vi "cm2nm_add_point_to_list.vi"(0 "SampleDataPoint":T1, 1 "SessionIndex":i32, 3 "Sample locations of Interest":refnum<vi>) -> (2 "sampleOf_interest_duplicate":refnum<vi>)   [LabVIEW 2011]
doc: "add_point_to_list \nadds a sample point to the table whose rows are the unique sample location and the collumns are the sessions. An X in the the row/col combination indicates the sample has been acquired in a particular session. A more complicated variation may be devised later.\n\nif the string associated with the location ID is unique then a new row for this sample will be added to the table and the row labels modified to include this. At this time no sorting will supported but could be added in future revisions.\n\nInputs\nReference to sample locations of Interest Table: reference to the table object on the top level front panel. Passed as a reference so the Row label array can be altered as well as the value of the table locations\n\nSampleDataPoint is the information about the current sample being added to the table. The necessary information is the Location Name/ID. That will be compared to the Row label strings to determine if it existed in prior sessions so it can be assigned to the same row or have a new row created for it.\n\nSessionIndex: number related the session of this data point to the collumn. It is the same index as that stored in the sample data base session lilst.\n\nSampleIndex: number of named samples in the table."
uses:
  cm2nm_coordinate_information_v2.ctl
panel:
  out "size(s)":i32[](array[numeric])
  out "Value":string[][](table)
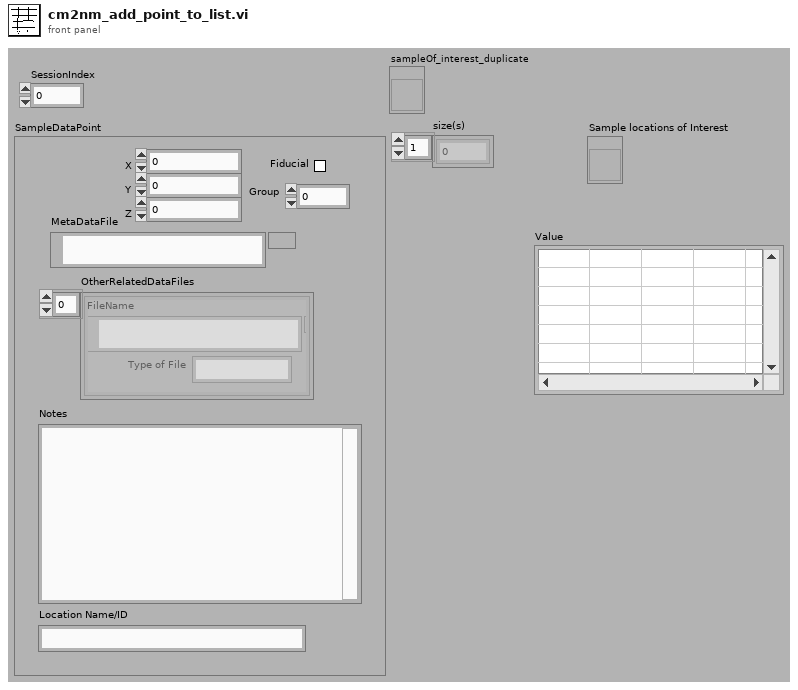
[diagram p1: front panel]
types:
  T1 = typedef "cm2nm_coordinate_information_v2.ctl" = cluster{"MetaDataFile":path, "X":dbl, "Y":dbl, "Z":dbl, "Group":i32, "Rotation":dbl[unit], "Fiducial":bool, "Magnification":dbl, "Working_Distance":dbl, "Notes":string, "Location Name/ID":string, "OtherRelatedDataFiles":cluster{"Type of File":string, "FileName":path}[], "Available":bool}
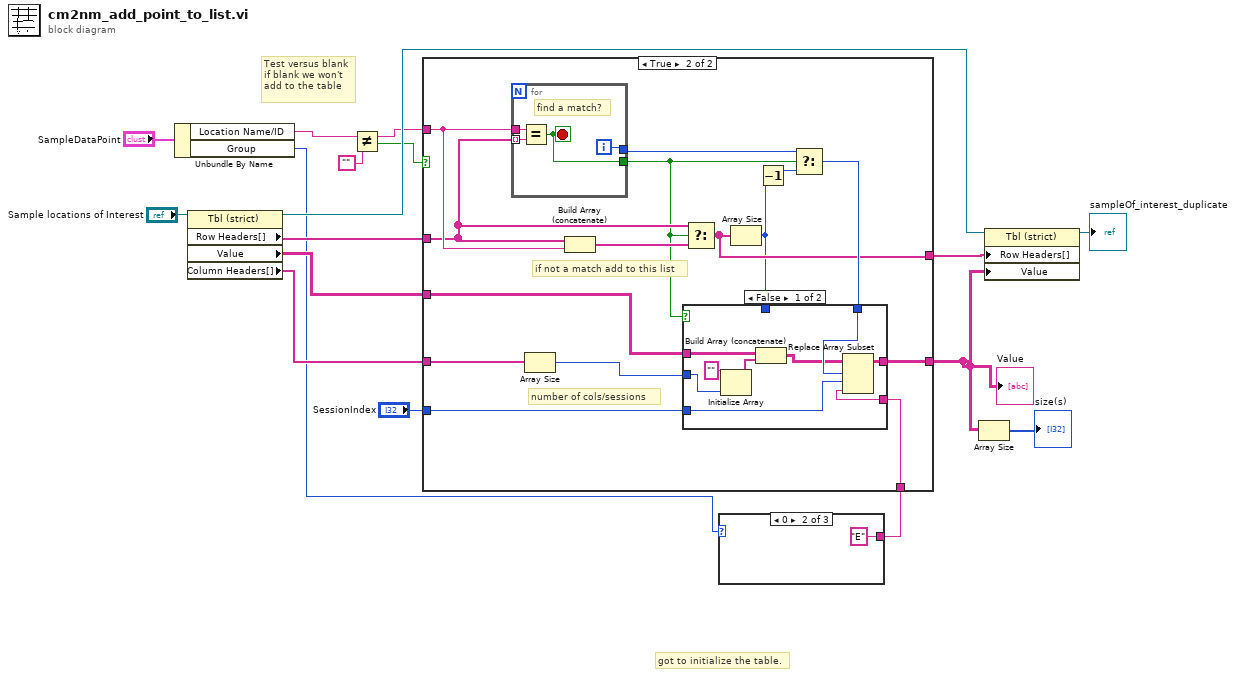
[diagram p0: block diagram]
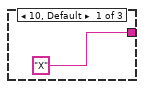
[diagram p2: hidden frame]
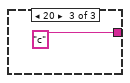
[diagram p3: hidden frame]
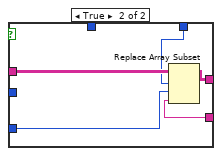
[diagram p5: hidden frame]
diagram:
  # "got to initialize the table."
  # "Test versus blank\nif blank we won't\nadd to the table"
  n1 = Unbundle By Name("SampleDataPoint") -> ("Location Name/ID"=w9:string, "Group"=w4:i32)
  n2 = property on="Property Node" class="Tbl (strict)"(reference="Sample locations of Interest") -> (reference out=w16:refnum<vi>, "Row Headers[]"=w13:string[], "Value"=w7:string[][], "Column Headers[]"=w6:string[])  [unwired: 1 in, 1 out]
  n3 = Not Equal?(x=w9, y="") -> (x != y?=w11:bool)
  n4 = case shown="0" w4 {
    tunnel: ["X" ("new element/subarray") "E" ("new element/subarray") "c" ("new element/subarray")] -> w3
    frame 10, Default {
    }
    frame 0 {
    }
    frame 20 {
    }
  }
  n5 = case shown="True" w11 {
    tunnel: w9 -> [_ w35]
    tunnel: "SessionIndex" -> [_ w34]
    tunnel: w13 -> [w21 w31]
    tunnel: [w21 w27] -> w14
    tunnel: w7 -> [w20 w23]
    tunnel: [w20 w30] -> w2
    tunnel: w6 -> [_ w25]
    tunnel: w3 -> [_ w22]
    frame False {
    }
    frame True {
      # "number of cols/sessions"
      # "if not a match add to this list"
      n6 = for {
        tunnel: w31 -> [w53] mode=indexing
        tunnel: w35 -> [w54]
        tunnel: [w51] -> w28
        tunnel: [w52] -> w32
        i -> [w52]
        stop <- w51 stop-if-true
        # "find a match?"
        n7 = Equal?(x=w54, y=w53) -> (x = y?=w51:bool)
      }
      n8 = Array Size(array=w25) -> (size(s)=w24:i32)
      n9 = Build Array (concatenate)(w31, w35) -> (w36:string[])
      n10 = Select(t=w31, s=w28, f=w36) -> (s? t:f=w27:string[])
      n11 = Array Size(array=w27) -> (size(s)=w26:i32)
      n12 = Decrement(x=w26) -> (x-1=w29:i32)
      n13 = Select(t=w32, s=w28, f=w29) -> (s? t:f=w33:i32)
      n14 = case shown="False" w28 {
        tunnel: w23 -> [w42 w50]
        tunnel: w33 -> [w45 w47]
        tunnel: w34 -> [w44 w49]
        tunnel: [w43 w48] -> w30
        tunnel: w24 -> [w40 _]
        tunnel: w26 -> [_ _]
        tunnel: w22 -> [w37 w46]
        frame False {
          n15 = Initialize Array("" ("new element/subarray"), w40) -> (w39:string[])
          n16 = Build Array (concatenate)(w42, w39) -> (w38:string[][])
          n17 = Replace Array Subset(array=w38, new element=w37, index (row)=w45, index (col)=w44) -> (w43:string[][])
        }
        frame True {
          n18 = Replace Array Subset(array=w50, new element=w46, index (row)=w47, index (col)=w49) -> (w48:string[][])
        }
      }
    }
  }
  "Value" <- w2
  n19 = Array Size(array=w2) -> (size(s)=→"size(s)":i32[])
  n20 = property on="Property Node" class="Tbl (strict)"(reference=w16, "Row Headers[]"=w14, "Value"=w2) -> (reference out=→"sampleOf_interest_duplicate":refnum<vi>)  [unwired: 1 in, 1 out]
